vi "Temperature and Pressure Monitor.vi"() -> ()   [LabVIEW 2013]
uses:
  <vilib>/Utility/miscctls.llb/LVPointTypeDef.ctl
  <vilib>/addons/database/_DB Variant To Data/Database Variant To Data.xnode
  <vilib>/addons/database/NI_Database_API.lvlib
panel:
  in  "Go":bool
  out "error out":errorcluster
  in  "error in (no error)":errorcluster
  out "Temperature (F)":dbl[](graph)
  out "Pressure (torr)":dbl[](graph)
  in  "Stop":bool
  out "Pressure (torr)":dbl
  out "Temperature (F)":dbl
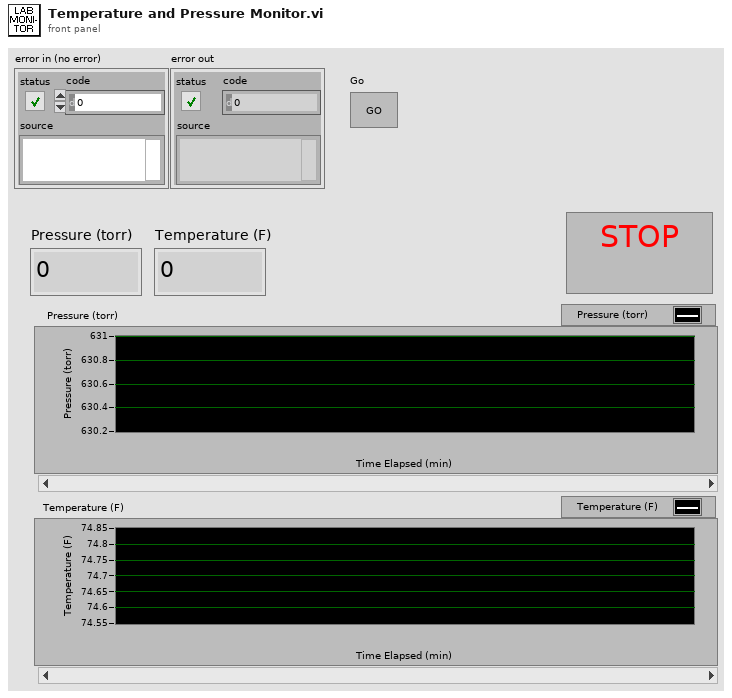
[diagram p1: front panel]
types:
  T1 = typedef "LVPointTypeDef.ctl" = cluster{"Horizontal":i16, "Vertical":i16}
  T2 = typedef "NI_Database_API.lvlib/Conn ObjectReference.ctl" = refnum<k1>
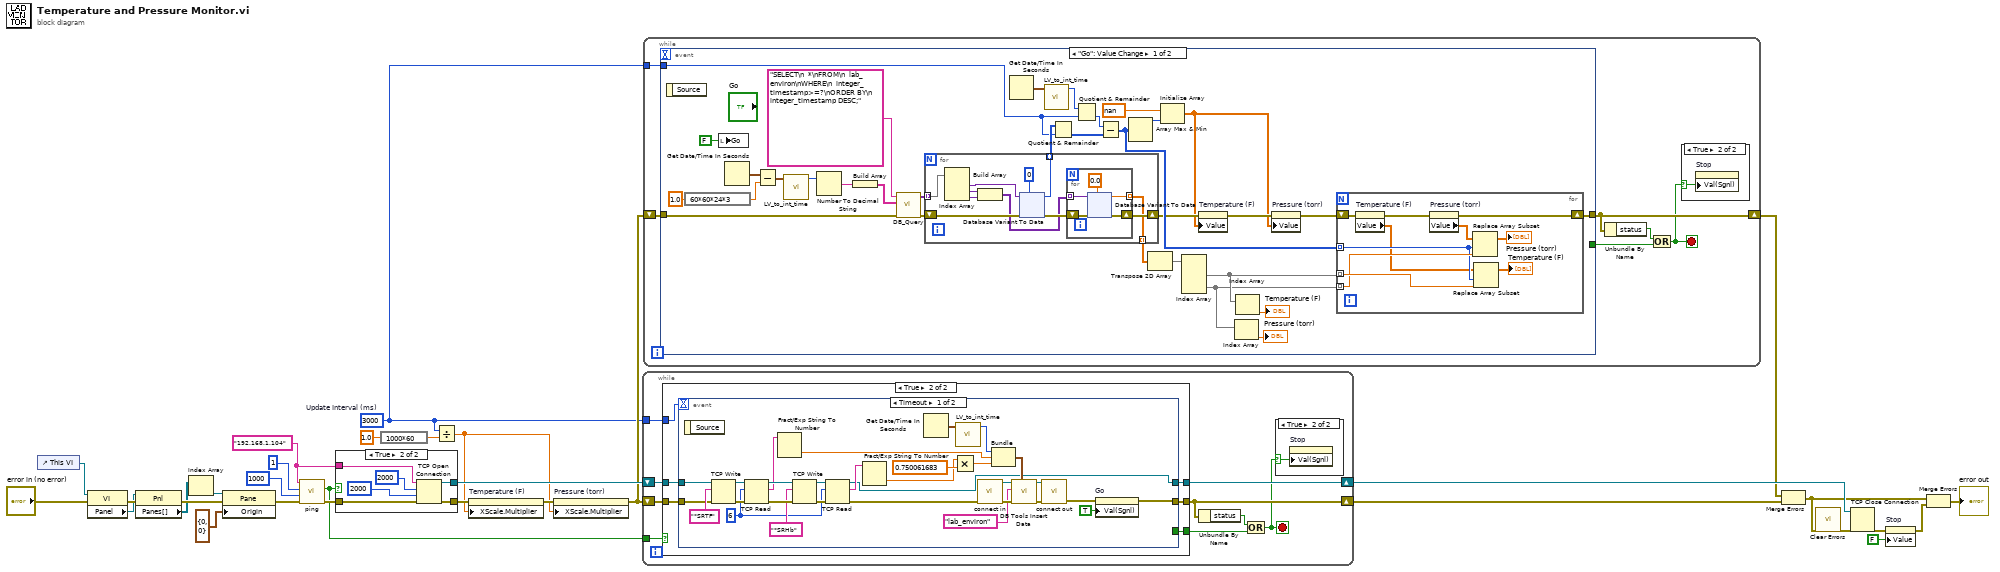
[diagram p0: block diagram]
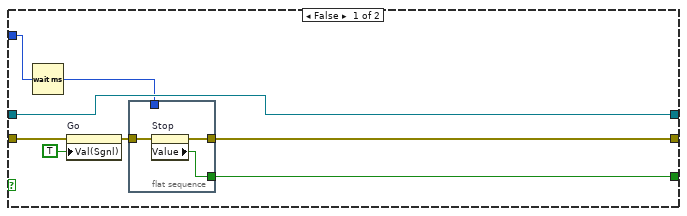
[diagram p2: hidden frame]
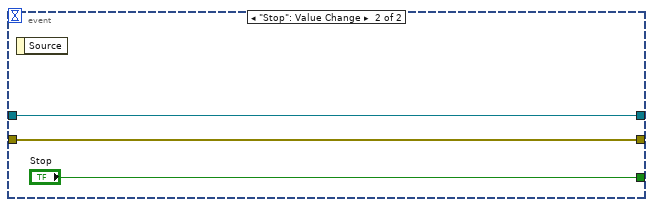
[diagram p3: hidden frame]
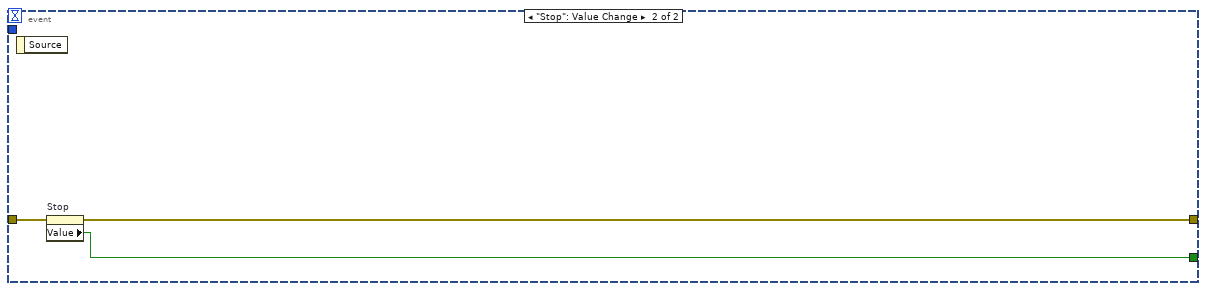
[diagram p6: hidden frame]
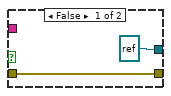
[diagram p7: hidden frame]
diagram:
  w4 = i64 3000  # Update Interval (ms)
  w8 = "192.168.1.104" ("host")
  n1 = control-ref of="This VI"() -> (w28:refnum<vi>)
  n2 = property class="VI"(reference=w28, error in="error in (no error)") -> (error out=w27:errorcluster, "Panel"=w26:refnum<vi>)  [unwired: 1 out]
  n3 = property class="Pnl"(reference=w26, error in=w27) -> (error out=w25:errorcluster, "Panes[]"=w24:refnum<vi>[])  [unwired: 1 out]
  n4 = Index Array(array=w24) -> (element=w23:refnum<vi>)  [unwired: 1 in]
  n5 = property class="Pane"(reference=w23, error in=w25, "Origin"=T1 {"Horizontal"=0, "Vertical"=0}) -> (error out=w21:errorcluster)  [unwired: 1 out]
  n6 = call "ping.vi"("error in"=w21, "timeout (ms)"=1000, "count"=1, "host"=w8) -> ("error out"=w29:errorcluster, "found?"=w11:bool)  [unwired: 5 in, 1 out]
  n7 = case shown="True" w11 {
    tunnel: [refnum<k5> refnum ("connection ID") w38] -> w19
    tunnel: [w32 w37] -> w5
    tunnel: w29 -> [w32 w35]
    tunnel: w8 -> [_ w34]
    frame False {
    }
    frame True {
      n8 = TCP Open Connection(address=w34, remote port or service name=i16 2000 ("Read Port"), timeout ms (60000)=2000, error in (no error)=w35) -> (connection ID=w38:refnum<k5>, error out=w37:errorcluster)  [unwired: 1 in]
    }
  }
  n9 = expression code="1000*60"(1.0) -> (w1:dbl)
  n10 = Divide(x=w4, y=w1) -> (x/y=w3:dbl)
  n11 = property on="Temperature (F)" class="WFGraph (strict)"(error in=w5, "XScale.Multiplier"=w3) -> (error out=w7:errorcluster)  [unwired: 1 in, 1 out]
  n12 = property on="Pressure (torr)" class="WFGraph (strict)"(error in=w7, "XScale.Multiplier"=w3) -> (error out=w6:errorcluster)  [unwired: 1 in, 1 out]
  n13 = while {
    shift-right: [w46] -> w16
    shift-left: w19 -> [w48]
    shift-right: [w45] -> w13
    shift-left: w6 -> [w47]
    tunnel: w4 -> [w41]
    tunnel: w11 -> [w40]
    stop <- w42 stop-if-true
    n14 = case shown="True" w40 {
      tunnel: w48 -> [w56 w65]
      tunnel: w47 -> [w52 w64]
      tunnel: [w56 w63] -> w46
      tunnel: [w50 w62] -> w45
      tunnel: [w55 w61] -> w43
      tunnel: w41 -> [w53 w60]
      frame False {
        n15 = Wait (ms)(milliseconds to wait=w53) -> (millisecond timer value=w49:u32)
        n16 = property on="Go" class="Bool (strict)"(error in=w52, "Val(Sgnl)"=TRUE ("Value (Signaling)")) -> (error out=w51:errorcluster)  [unwired: 1 in, 1 out]
        n17 = flat-sequence {
          tunnel: [w59] -> w55
          tunnel: w51 -> [w58]
          tunnel: [w57] -> w50
          tunnel: w49 -> [_]
          frame #0 {
            n18 = property on="Stop" class="Bool (strict)"(error in=w58) -> (error out=w57:errorcluster, "Value"=w59:bool)  [unwired: 1 in, 1 out]
          }
        }
      }
      frame True {
        n19 = event shown="[0] Timeout" {
          selector: _ -> [_ _]
          dyn-events: _ -> [_ _]
          timeout: w60 -> [_ _]
          tunnel: w65 -> [w95 w97]
          tunnel: w64 -> [w92 w98]
          tunnel: [w66 w97] -> w63
          tunnel: [w75 w98] -> w62
          tunnel: [_ "Stop"] -> w61
          event Timeout {
            w81 = 6 ("bytes to read")
            n20 = event-data() -> ()  [unwired: 1 in, 1 out]
            n21 = TCP Write(connection ID=w95, data in="*SRTF", error in (no error)=w92) -> (connection ID out=w94:refnum<k5>, error out=w91:errorcluster)  [unwired: 1 in, 1 out]
            n22 = TCP Read(connection ID=w94, bytes to read=w81, error in (no error)=w91) -> (connection ID out=w87:refnum<k5>, data out=w85:string, error out=w88:errorcluster)  [unwired: 2 in]
            n23 = Fract/Exp String To Number(string=w85) -> (number=w77:dbl)  [unwired: 3 in, 1 out]
            n24 = TCP Write(connection ID=w87, data in="*SRHb", error in (no error)=w88) -> (connection ID out=w89:refnum<k5>, error out=w90:errorcluster)  [unwired: 1 in, 1 out]
            n25 = TCP Read(connection ID=w89, bytes to read=w81, error in (no error)=w90) -> (connection ID out=w66:refnum<k5>, data out=w84:string, error out=w67:errorcluster)  [unwired: 2 in]
            n26 = Fract/Exp String To Number(string=w84) -> (number=w82:dbl)  [unwired: 3 in, 1 out]
            n27 = Get Date/Time In Seconds() -> (seconds since 1Jan1904=w80:timestamp)
            n28 = Multiply(x=w82, y=0.750061683) -> (x*y=w76:dbl)
            n29 = call "LV_to_int_time.vi"("Time Stamp"=w80) -> ("Integer Time"=w78:i64)  [unwired: 8 in, 1 out]
            n30 = call "connect in.vi"("error in (no error)"=w67) -> ("error out"=w73:errorcluster, "Database Connection"=w72:T2)  [unwired: 7 in]
            n31 = Bundle("Integer Time"=w78, w77, w76) -> (w79:cluster{"Integer Time":i64, dbl, dbl})  [unwired: 1 in]
            n32 = call <vilib>:"DB Tools Insert Data.vi"("data"=w79, "error in (no error)"=w73, "table"="lab_environ" ("string"), "connection reference"=w72) -> ("error out"=w74:errorcluster, "connection reference out"=w71:T2)  [unwired: 6 in]
            n33 = call "connect out.vi"("error in (no error)"=w74, "connection reference"=w71) -> ("error out"=w69:errorcluster)  [unwired: 9 in]
            n34 = property on="Go" class="Bool (strict)"(error in=w69, "Val(Sgnl)"=TRUE ("Value (Signaling)")) -> (error out=w75:errorcluster)  [unwired: 1 in, 1 out]
          }
          event "Stop": Value Change {
            n35 = event-data() -> ()  [unwired: 1 in, 1 out]
          }
        }
      }
    }
    n36 = Unbundle By Name(w45) -> ("status"=w44:bool)
    n37 = Or(x=w44, y=w43) -> (x .or. y?=w42:bool)
    n38 = case shown="True" w42 {
      selector: w42 -> [_ w99]
      frame False {
      }
      frame True {
        n39 = property on="Stop" class="Bool (strict)"("Val(Sgnl)"=w99) -> ()  [unwired: 2 in, 2 out]
      }
    }
  }
  n40 = while {
    shift-right: [w103] -> w14
    shift-left: w6 -> [w105]
    tunnel: w4 -> [w100]
    stop <- w101 stop-if-true
    n41 = event shown="[0] \"Go\": Value Change" {
      selector: _ -> [_ _]
      dyn-events: _ -> [_ _]
      timeout: _ -> [_ _]
      tunnel: [w111 w230] -> w103
      tunnel: w105 -> [w113 w229]
      tunnel: [_ w231] -> w102
      tunnel: w100 -> [w112 _]
      event "Go": Value Change {
        n42 = event-data() -> ()  [unwired: 1 in, 1 out]
        n43 = expression code="60*60*24*3"(1.0) -> (w120:dbl)
        n44 = local write "Go"(FALSE ("Go")) -> ()
        n45 = Get Date/Time In Seconds() -> (seconds since 1Jan1904=w138:timestamp)
        n46 = Subtract(x=w138, y=w120) -> (x-y=w133:timestamp)
        n47 = call "LV_to_int_time.vi"("Time Stamp"=w133) -> ("Integer Time"=w137:i64)  [unwired: 8 in, 1 out]
        n48 = Number To Decimal String(number=w137) -> (decimal integer string=w136:string)  [unwired: 1 in]
        n49 = Build Array(w136) -> (w135:string[])
        n50 = call "DB_Query.vi"("error in (no error)"=w113, "Parameters"=w135, "Parameterized Query"="SELECT\n  *\nFROM\n  lab_environ\nWHERE\n  integer_timestamp>=?\nORDER BY\n  integer_timestamp DESC;") -> ("error out"=w132:errorcluster, "Results"=w131:variant[][])  [unwired: 6 in, 1 out]
        n51 = for {
          shift-right: [w159] -> w115
          shift-left: w132 -> [w156]
          tunnel: [w158] -> w117 mode=indexing
          tunnel: [w157] -> w130 mode=indexing
          tunnel: w131 -> [w153] mode=indexing
          n52 = Index Array(array=w153) -> (element #1=w150:variant, element #2=w152:variant, element #3=w151:variant)  [unwired: 3 in]
          n53 = Build Array(w152, w151) -> (w149:variant[])
          n54 = xnode "Database Variant To Data"("database variant"=w150, "error in (no error)"=w156, "type"=i64 0) -> ("data"=w157:i64, "error out"=w155:errorcluster)
          n55 = for {
            shift-right: [w193] -> w159
            shift-left: w155 -> [w196]
            tunnel: w149 -> [w194] mode=indexing
            tunnel: [w192] -> w158 mode=indexing
            n56 = xnode "Database Variant To Data"("database variant"=w194, "error in (no error)"=w196, "type"=0.0) -> ("data"=w192:dbl, "error out"=w193:errorcluster)
          }
        }
        n57 = Get Date/Time In Seconds() -> (seconds since 1Jan1904=w128:timestamp)
        n58 = call "LV_to_int_time.vi"("Time Stamp"=w128) -> ("Integer Time"=w126:i64)  [unwired: 8 in, 1 out]
        n59 = Quotient & Remainder(x=w130, y=w112) -> (floor(x/y)=w129:i64[])  [unwired: 1 out]
        n60 = Quotient & Remainder(x=w126, y=w112) -> (floor(x/y)=w127:i64)  [unwired: 1 out]
        n61 = Subtract(x=w127, y=w129) -> (x-y=w125:i64[])
        n62 = Array Max & Min(array=w125) -> (max value=w118:i64)  [unwired: 3 out]
        n63 = Transpose 2D Array(2D array=w117) -> (transposed array=w107:dbl[][])
        n64 = Initialize Array(nan, w118) -> (w114:dbl[])
        n65 = Index Array(array=w107) -> (element #1=w124:dbl[], element #2=w122:dbl[])  [unwired: 4 in]
        n66 = property on="Temperature (F)" class="WFGraph (strict)"(error in=w115, "Value"=w114) -> (error out=w116:errorcluster)  [unwired: 1 in, 1 out]
        n67 = Index Array(array=w122) -> (element=→"Pressure (torr)":dbl)  [unwired: 1 in]
        n68 = Index Array(array=w124) -> (element=→"Temperature (F)":dbl)  [unwired: 1 in]
        n69 = property on="Pressure (torr)" class="WFGraph (strict)"(error in=w116, "Value"=w114) -> (error out=w108:errorcluster)  [unwired: 1 in, 1 out]
        n70 = for {
          tunnel: w124 -> [w148] mode=indexing
          tunnel: w125 -> [w144] mode=indexing
          tunnel: w122 -> [w145] mode=indexing
          shift-right: [w139] -> w111
          shift-left: w108 -> [w140]
          n71 = property on="Temperature (F)" class="WFGraph (strict)"(error in=w140) -> (error out=w142:errorcluster, "Value"=w141:dbl[])  [unwired: 1 in, 1 out]
          n72 = property on="Pressure (torr)" class="WFGraph (strict)"(error in=w142) -> (error out=w139:errorcluster, "Value"=w143:dbl[])  [unwired: 1 in, 1 out]
          n73 = Replace Array Subset(array=w143, new element=w145, index=w144) -> (→"Pressure (torr)":dbl[])
          n74 = Replace Array Subset(array=w141, new element=w148, index=w144) -> (→"Temperature (F)":dbl[])
        }
      }
      event "Stop": Value Change {
        n75 = event-data() -> ()  [unwired: 1 in, 1 out]
        n76 = property on="Stop" class="Bool (strict)"(error in=w229) -> (error out=w230:errorcluster, "Value"=w231:bool)  [unwired: 1 in, 1 out]
      }
    }
    n77 = Unbundle By Name(w103) -> ("status"=w104:bool)
    n78 = Or(x=w104, y=w102) -> (x .or. y?=w101:bool)
    n79 = case shown="True" w101 {
      selector: w101 -> [_ w106]
      frame False {
      }
      frame True {
        n80 = property on="Stop" class="Bool (strict)"("Val(Sgnl)"=w106) -> ()  [unwired: 2 in, 2 out]
      }
    }
  }
  n81 = Merge Errors(w14, w13) -> (w9:errorcluster)
  n82 = call <vilib>:"Clear Errors.vi"("error in (no error)"=w9) -> ("error out"=w15:errorcluster)  [unwired: 6 in]
  n83 = TCP Close Connection(connection ID=w16, error in (no error)=w15) -> (error out=w18:errorcluster)  [unwired: 1 in, 1 out]
  n84 = property on="Stop" class="Bool (strict)"(error in=w18, "Value"=FALSE ("Stop")) -> (error out=w10:errorcluster)  [unwired: 1 in, 1 out]
  n85 = Merge Errors(w9, w10) -> (→"error out":errorcluster)
